vi "Periodic Tasks.vi"(8 "error in":errorcluster) -> ()   [LabVIEW 2015]
doc: "This VI runs in parallel to other tasks. It can contain as many user-defined periodic loops as you need. These can carry out PID or other sorts of timed response."
uses:
  <vilib>/Rock Robotics/WPI/Utilities/WPI_GetSetVariantRefNum.vi
  Robot Global Data.vi
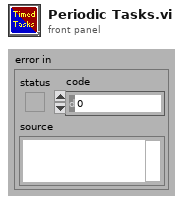
[diagram p1: front panel]
types:
  T1 = typedef "WPI_JoystickDevRef.ctl" = cluster{"Device":T2}
  T2 = typedef "WPI_JoystickDeviceEnum.ctl" = enum16{"USB 0", "USB 1", "USB 2", "USB 3", "USB 4", "USB 5"}
  T3 = typedef "WPI_RobotDriveDevRef.ctl" = cluster{"DevStatus":errorcluster, "Motors[]":T4[], "Square Inputs":bool, "Max Output":dbl}
  T4 = typedef "WPI_MotorControlDeviceRef.ctl" = cluster{"DeviceStatus":errorcluster, "Type":T5, "PWM":cluster{"PWM Channel":T6, "DeadBand":T7}, "CAN":cluster{"Device Number":u8, "Control Mode":T8, "Semaphore":T9, "Max Vout":dbl, "TalonSRX Control Mode":T10}, "Invert":bool}
  T5 = typedef "WPI_MotorControlType.ctl" = enum16{"PWM", "CAN", "CANTalonSRX"}
  T6 = typedef "FPGA_DIOPWMChannel.ctl" = enum8{"PWM 0", "PWM 1", "PWM 2", "PWM 3", "PWM 4", "PWM 5", "PWM 6", "PWM 7", "PWM 8", "PWM 9", "PWM MXP 0", "PWM MXP 1", "PWM MXP 2", "PWM MXP 3", "PWM MXP 4", "PWM MXP 5", "PWM MXP 6", "PWM MXP 7", "PWM MXP 8", "PWM MXP 9", "Invalid"}
  T7 = typedef "WPI_PWMDeadband.ctl" = cluster{"Name":string, "maxPositivePwm":i32, "minPositivePwm":i32, "centerPwm":i32, "maxNegativePwm":i32, "minNegativePwm":i32, "angularRange":u16}
  T8 = typedef "WPI_CANJaguar_ControlMode.ctl" = enum8{"Percent VBus", "Current", "Speed", "Position", "Voltage"}
  T9 = typedef "Semaphore RefNum" = refnum<k1>
  T10 = typedef "WPI_CANTalonSRX_APIControlMode.ctl" = enum8{"Percent VBus", "Speed", "Position", "Slave", "Unchanged / Invalid", "Voltage Compensation", "Current", "Motion Profile"}
  T11 = cluster{"JoystickDevRef":T1, "RobotDriveDevRef":T3}
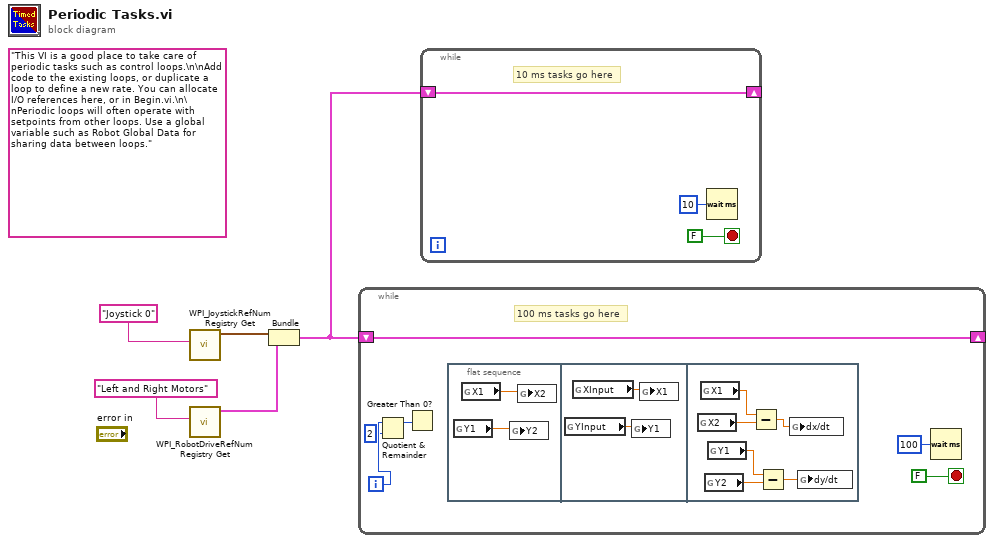
[diagram p0: block diagram]
diagram:
  (unwired) "This VI is a good place to take care of periodic tasks such as control loops.\n\nAdd code to the existing loops, or duplicate a loop to define a new rate. You can allocate I/O references here, or in Begin.vi.\n\nPeriodic loops will often operate with setpoints from other loops. Use a global variable such as Robot Global Data for sharing data between loops."
  n1 = call <vilib>:"WPI_JoystickRefNum Registry Get.vi"("refnum name"="Joystick 0") -> ("JoystickDevRef"=w3:T1)  [unwired: 1 in, 9 out]
  n2 = call <vilib>:"WPI_RobotDriveRefNum Registry Get.vi"("refnum name"="Left and Right Motors") -> ("RobotDriveDevRef"=w2:T3)  [unwired: 1 in, 9 out]
  n3 = Bundle("JoystickDevRef"=w3, "RobotDriveDevRef"=w2) -> (w1:T11)  [unwired: 1 out]
  n4 = while {
    shift-right: [w9] -> _
    shift-left: w1 -> [w9]
    i -> [w8]
    stop <- FALSE stop-if-true
    # "100 ms tasks go here"
    n5 = Quotient & Remainder(x=w8, y=2) -> (x-y*floor(x/y)=w6:i32)  [unwired: 1 out]
    n6 = Greater Than 0?(x=w6) -> ()  [unwired: 1 out]
    n7 = flat-sequence {
      frame #0 {
        n8 = global read "Robot Global Data.vi" "Y1"() -> (w12:dbl)
        n9 = global read "Robot Global Data.vi" "X1"() -> (w13:dbl)
        n10 = global write "Robot Global Data.vi" "Y2"(w12) -> ()
        n11 = global write "Robot Global Data.vi" "X2"(w13) -> ()
      }
      frame #1 {
        n12 = global read "Robot Global Data.vi" "YInput"() -> (w14:dbl)
        n13 = global read "Robot Global Data.vi" "XInput"() -> (w15:dbl)
        n14 = global write "Robot Global Data.vi" "Y1"(w14) -> ()
        n15 = global write "Robot Global Data.vi" "X1"(w15) -> ()
      }
      frame #2 {
        n16 = global read "Robot Global Data.vi" "X2"() -> (w20:dbl)
        n17 = global read "Robot Global Data.vi" "X1"() -> (w21:dbl)
        n18 = global read "Robot Global Data.vi" "Y2"() -> (w18:dbl)
        n19 = global read "Robot Global Data.vi" "Y1"() -> (w19:dbl)
        n20 = Subtract(x=w21, y=w20) -> (x-y=w16:dbl)
        n21 = Subtract(x=w19, y=w18) -> (x-y=w17:dbl)
        n22 = global write "Robot Global Data.vi" "dx/dt"(w16) -> ()
        n23 = global write "Robot Global Data.vi" "dy/dt"(w17) -> ()
      }
    }
    n24 = Wait (ms)(milliseconds to wait=u32 100) -> ()  [unwired: 1 out]
  }
  n25 = while {
    shift-right: [w22] -> _
    shift-left: w1 -> [w22]
    stop <- FALSE stop-if-true
    # "10 ms tasks go here"
    n26 = Wait (ms)(milliseconds to wait=u32 10) -> ()  [unwired: 1 out]
  }
